vi "LED-Ctl2Ind.vi"(2 "Action 2":T3 caption="Action", 3 "Container State":T1, 4 "Display State In 2":T2 caption="State" {"Flags" format="%x"}) -> (0 "Action":T3, 1 "Display State In":T2 caption="State" {"Flags" format="%x"})   [LabVIEW 2010, in "LED Display.xctl"]
uses:
  LED Display.xctl
  <vilib>/_xctls/Action.ctl
  LED-State.ctl
  <vilib>/_xctls/Container State.ctl
  <vilib>/_xctls/XControlSupport.lvlib
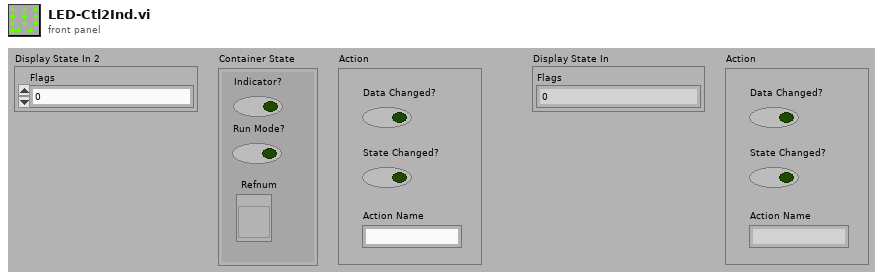
[diagram p1: front panel]
types:
  T1 = typedef "XControlSupport.lvlib/Container State.ctl" = cluster{"Indicator?":bool, "Run Mode?":bool, " Refnum":refnum<vi>}
  T2 = typedef "LED Display.xctl/LED-State.ctl" = cluster{"Flags":u64}
  T3 = typedef "XControlSupport.lvlib/Action.ctl" = cluster{"Data Changed?":bool, "State Changed?":bool, "Action Name":string}
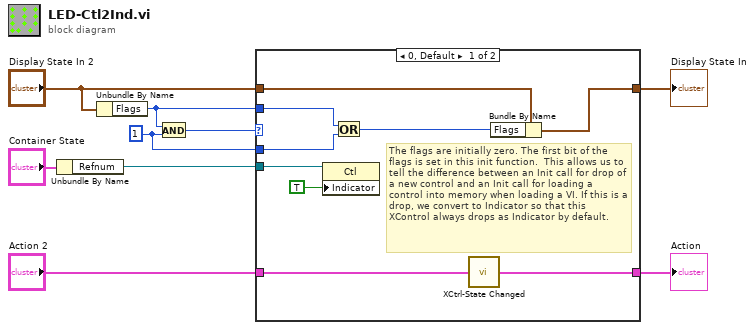
[diagram p0: block diagram]
diagram:
  w7 = u64 1 ("Flags")
  n1 = Unbundle By Name("Container State") -> ("Refnum"=w3:refnum<vi>)
  n2 = Unbundle By Name("Display State In 2") -> ("Flags"=w6:u64)
  n3 = And(x=w6, y=w7) -> (x .and. y?=w2:u64)
  n4 = case shown="0, Default" w2 {
    tunnel: w3 -> [w18 _]
    tunnel: [w12 w20] -> w5
    tunnel: "Display State In 2" -> [w14 w20]
    tunnel: w6 -> [w16 _]
    tunnel: w7 -> [w15 _]
    tunnel: "Action 2" -> [w10 w19]
    tunnel: [w11 w19] -> w9
    frame 0, Default {
      # "The flags are initially zero. The first bit of the flags is set in this init function.  This allows us to tell the difference between an Init call for drop of a new control and an Init call for loading a control into memory when loading a VI. If this is a drop, we convert to Indicator so that this XControl always drops as Indicator by default."
      n5 = property class="Ctl"(reference=w18, "Indicator"=TRUE) -> ()  [unwired: 1 in, 2 out]
      n6 = Or(x=w16, y=w15) -> (x .or. y?=w13:u64)
      n7 = call "XCtrl-State Changed.vi"("Action"=w10) -> ("Action 2"=w11:T3)
      n8 = Bundle By Name(cluster=w14, "Flags"=w13) -> (w12:T2)
    }
    frame 1 {
    }
  }
  "Action" <- w9
  "Display State In" <- w5
